vi "SDT_GenerateInfoBlock.vi"(4 "ActiveModule":string[](array[string]), 6 "Contents":string="LV SDT-Data", 7 "FileType":T1=1 items=["non-Fifo"=1, "Fifo"=2, "FifoImage"=3], 9 "FileID":string="SPC FCS Data File", 10 "adc_re[dig]":u32=256, 11 "FilenameNoExtension":string) -> (3 "Info Block":string)   [LabVIEW 2019]
doc: "This VI is a SubVI to SDT_WriteFile.vi. and SPCWriteSETfoSPC.vi.\nIt formats the Info Block ready to be written to file. \nFor a description of the *.sdt file format see: SPC_data_file_structure.h\n\ninfo@becker-hickl.com"
uses:
  SPC_Controls/FileType.ctl
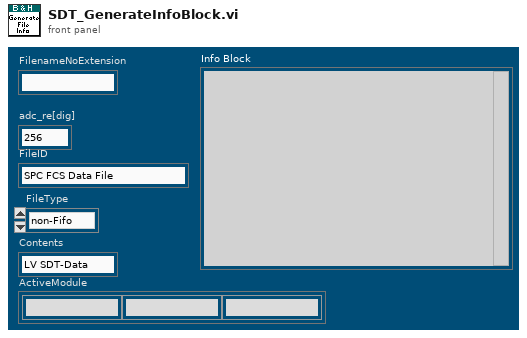
[diagram p1: front panel]
types:
  T1 = typedef "FileType.ctl" = u16
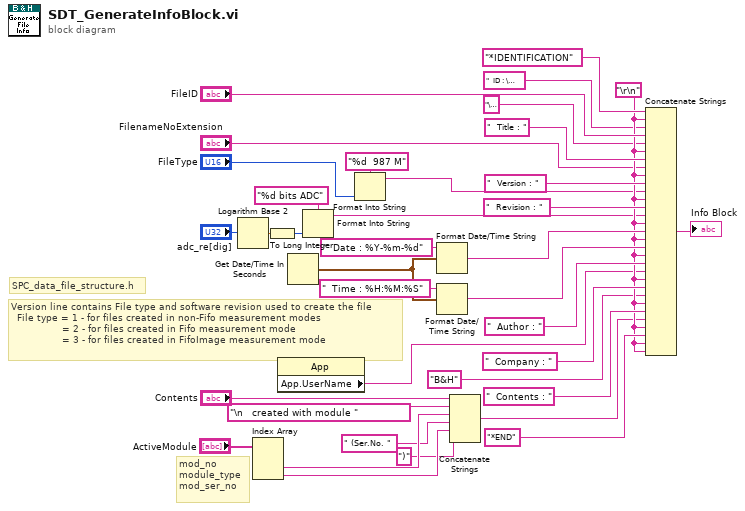
[diagram p0: block diagram]
diagram:
  w22 = "\r\n"
  # "mod_no\nmodule_type\nmod_ser_no"
  # "SPC_data_file_structure.h"
  # "Version line contains File type and software revision used to create the file \n  File type = 1 - for files created in non-Fifo measurement modes\n                 = 2 - for files created in Fifo measurement mode\n                 = 3 - for files created in FifoImage measurement mode"
  n1 = Logarithm Base 2(1:"adc_re[dig]") -> (0:w20:dbl)
  n2 = Index Array(array="ActiveModule") -> (element #2=w5:string, element #3=w3:string)  [unwired: 3 in, 1 out]
  n3 = To Long Integer(number=w20) -> (32bit integer=w21:i32)
  n4 = property class="App"() -> ("App.UserName"=w1:string)  [unwired: 2 in, 2 out]
  n5 = Get Date/Time In Seconds() -> (seconds since 1Jan1904=w28:timestamp)
  n6 = Format Into String(format string="%d bits ADC", w21) -> (resulting string=w16:string)  [unwired: 2 in, 1 out]
  n7 = Format Into String(format string="%d  987 M" ("Version"), "FileType") -> (resulting string=w9:string)  [unwired: 2 in, 1 out]
  n8 = Format Date/Time String(time format string (%c)="  Date : %Y-%m-%d", seconds (now)=w28) -> (date/time string=w31:string)  [unwired: 1 in]
  n9 = Format Date/Time String(time format string (%c)="  Time : %H:%M:%S", seconds (now)=w28) -> (date/time string=w29:string)  [unwired: 1 in]
  n10 = Concatenate Strings("Contents", "\n   created with module " ("string"), w5, " (Ser.No. " ("string"), w3, ")" ("string")) -> (w7:string)
  n11 = Concatenate Strings("*IDENTIFICATION", w22, "  ID : \u0004" ("FileID"), "FileID", "\u0004" ("string"), w22, "  Title : ", "FilenameNoExtension", w22, "  Version : ", w9, w22, "  Revision : ", w16, w22, w31, w22, w29, w22, "  Author : ", w1, w22, "  Company : ", "B&H" ("Company"), w22, "  Contents : ", w7, w22, "*END", w22, w22) -> (→"Info Block":string)
